vi "TSM SSC DAQmx Read (Analog 1D Wfm) System Pin.vi"(0 "DAQ TSM in":T1, 5 "Samples to read":i32=-1, 11 "error in":errorcluster) -> (4 "DAQ TSM Out":T1, 6 "System-Pin Waveforms Out":waveform(dbl), 15 "error out":errorcluster)   [LabVIEW 2020]
doc: "Reads one or more waveforms from a task that contains one or more analog input channels. The data will be ordered based on the SSC order."
uses:
  Pin Map/TSM DAQmx Multi-Task.ctl
  <vilib>/NI_TestStand_SemiconductorModule/NI_TestStand_Semiconductor_Module.lvlibp/PinMap/PinQueryContext/MultiplePinMultipleSessionQueryContext/MultiplePinMultipleSessionQueryContext.lvclass
  Pin Map/SSC DAQmx.ctl
  <vilib>/DAQmx/read.llb/DAQmx Read (Analog Wfm 1Chan NSamp).vi
  <vilib>/DAQmx/miscellaneous.llb/DAQmx Fill In Error Info.vi
  <resource>/objmgr/daqmx.rc
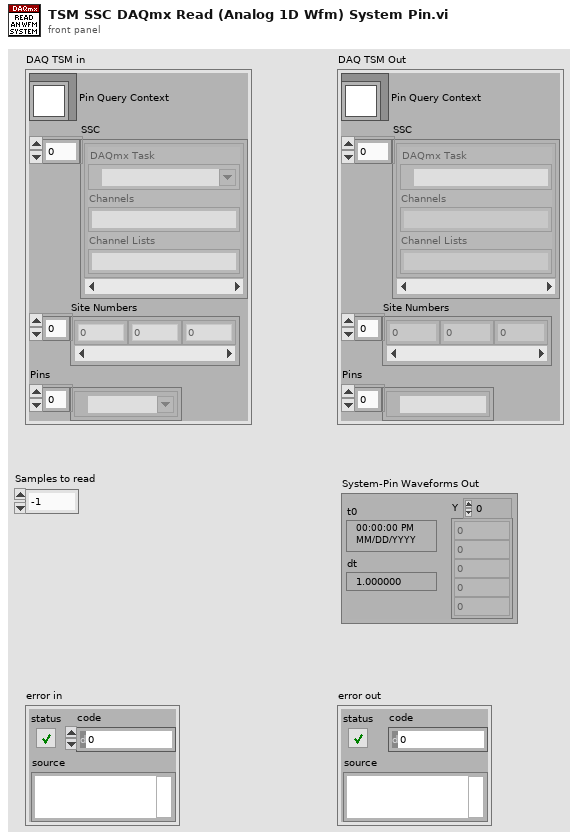
[diagram p1: front panel]
types:
  T1 = typedef "TSM DAQmx Multi-Task.ctl" = cluster{"Pin Query Context":refnum<class "MultiplePinMultipleSessionQueryContext.lvclass">, "SSC":T2[], "Site Numbers":i32[], "Pins":tag[]}
  T2 = typedef "SSC DAQmx.ctl" = cluster{"DAQmx Task ":refnum<k21>, "Channels":string, "Channel Lists":string}
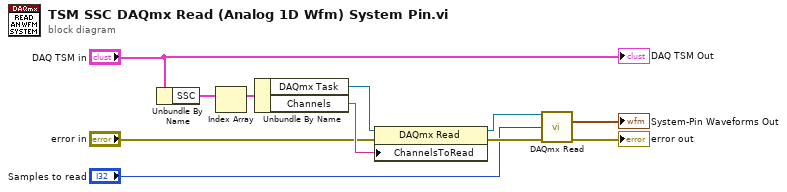
[diagram p0: block diagram]
diagram:
  n1 = Unbundle By Name("DAQ TSM in") -> ("SSC"=w5:T2[])
  n2 = Index Array(array=w5) -> (element=w6:T2)  [unwired: 1 in]
  n3 = Unbundle By Name(w6) -> ("DAQmx Task"=w8:refnum<k21>, "Channels"=w9:string)
  n4 = property class="DAQmx Read"(reference=w8, error in="error in", "ChannelsToRead"=w9) -> (reference out=w7:refnum<k21>, error out=w10:errorcluster)
  n5 = call-poly <vilib>:"DAQmx Read.vi"("task/channels in"=w7, "number of samples per channel"="Samples to read", "error in"=w10) -> ("data"=→"System-Pin Waveforms Out":waveform(dbl), "error out"=→"error out":errorcluster)  [unwired: 10 in, 1 out]
  "DAQ TSM Out" <- "DAQ TSM in"
